vi "Extended Peripherals_labserver_ed.vi"(2 "error in (no error)":errorcluster, 4 "Command In":string) -> (0 "error out (no error)":errorcluster, 1 "DataOut":string)   [LabVIEW 2011]
doc: "Extended Peripherals\n\nThis vi will contain extended functionality not fitting in the regular instrumentation, such as sets and resets.\n\nCommand In:\n0 Delay.\n3 Reset ALL!"
uses:
  Server_Globals.vi
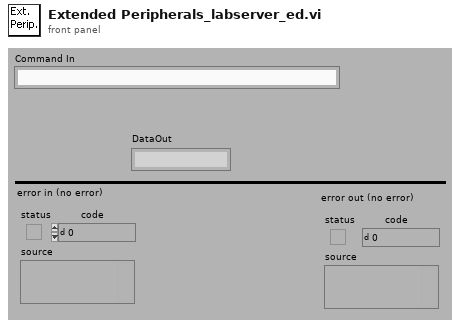
[diagram p1: front panel]
types:
  T1 = cluster{"I/O Settings":u64[], "Instrument Handle":cluster{"5402":refnum<k15>, " 5112":refnum<k15>, "4072":refnum<k15>, "USB":refnum<visa-resource-name>, "4110":refnum<k15>}, "Logfile":refnum<file>, "Log Level":i8, "Clear":i32[], "OS Set":cluster{"instrument handle out":refnum<k15>, "remaining string":string, "Settings":cluster{"Horizontal Conf.":cluster{"Min. Sample rate":dbl, "Reference position":dbl, "Record Length":i16}, "Channel A":cluster{"Enable":bool, "Vertical coupling":dbl, "Vertical range":dbl, "Vertical offset":dbl, "Probe attenuation":dbl}, "Channel B":cluster{"Enable":bool, "Vertical coupling":dbl, "Vertical range":dbl, "Vertical offset":dbl, "Probe attenuation":dbl}, "Trigger":cluster{"Source":enum8{"channel 1", "channel 2", "Imediate", "External trigger"}, "Slope":enum8{"Positive", "Negative"}, "Coupling":enum8{"AC", "DC"}, "Level":dbl, "Holdoff":dbl, "Delay":dbl, " Timeout":dbl, " Mode":enum8{"Normal", "Auto", "Auto Level"}}, "Measurements":cluster{"Measurement 1, Channel":enum8{"Channel 1", "Channel 2", "Channel 3", "Channel 4"}, "Measurement 1, Selection":u16, "Measurement 2, Channel":enum8{"Channel 1", "Channel 2", "Channel 3", "Channel 4"}, "Measurement 2,  Selection":u16, "Measurement 3, Channel":enum8{"Channel 1", "Channel 2", "Channel 3", "Channel 4"}, "Measurement 3, Selection 3":u16}}}, "DC Power Supply":cluster{"0":refnum<k15>, "1":refnum<k15>, "2":refnum<k15>, "3":refnum<k15>, "4":refnum<k15>}, "USB Interface":cluster{"0":refnum<visa-resource-name>, "1":refnum<visa-resource-name>, "2":refnum<visa-resource-name>, "3":refnum<visa-resource-name>, "4":refnum<visa-resource-name>}, "Function Generator":cluster{"0":refnum<k15>, "1":refnum<k15>, "2":refnum<k15>, "3":refnum<k15>, "4":refnum<k15>}, "Digital Multimeter":cluster{"0":refnum<k15>, "1":refnum<k15>, "2":refnum<k15>, "3":refnum<k15>, "4":refnum<k15>}, "Digital Osciliscope":cluster{"0":refnum<k15>, "1":refnum<k15>, "2":refnum<k15>, "3":refnum<k15>, "4":refnum<k15>}, "To M Server":string, "Adres":string[][], "Matrix version":string, "MD5":string, "Digital Multimeter Card 2":cluster{"0":string, "1":string, "2":string, "3":string, "4":string}}
  T2 = cluster{"Global":cluster{"Port":i32, "Reset Time":i32, "Maximum Delay":i32}, "Instrument Adress":cluster{"FGEN":string, "DC Power":string, "OSC":string, "USB":string, "DMM":string}, "Log":cluster{"Log Level":u32, "Log File":path}, "Digital Multimeter":cluster{"0":string, "1":string, "2":string, "3":string, "4":string}, "Function Generator":cluster{"0":string, "1":string, "2":string, "3":string, "4":string}, "Digital Osciliscope":cluster{"0":string, "1":string, "2":string, "3":string, "4":string}, "DC Power Supply":cluster{"0":string, "1":string, "2":string, "3":string, "4":string}, "USB Interface":cluster{"0":string, "1":string, "2":string, "3":string, "4":string}, "Components type":cluster{"Components type":string, "Components list":string}, "Matrix version":string, "Digital Multimeter Card 2":cluster{"0":string, "1":string, "2":string, "3":string, "4":string}}
  T3 = cluster{"0":refnum<k15>, "1":refnum<k15>, "2":refnum<k15>, "3":refnum<k15>, "4":refnum<k15>}
  T4 = cluster{"[0]":refnum<k15>, "[1]":refnum<k15>, "[2]":refnum<k15>, "[3]":refnum<k15>, "[4]":refnum<k15>}
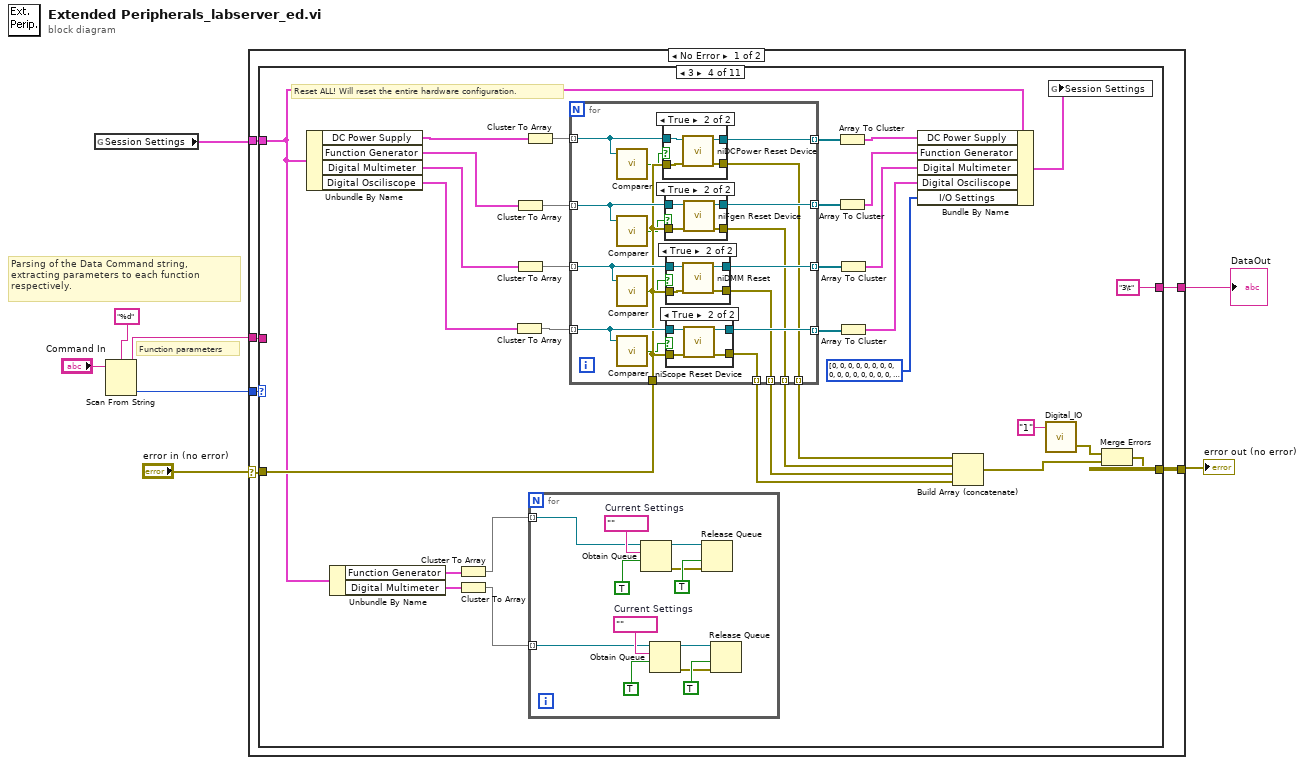
[diagram p0: block diagram]
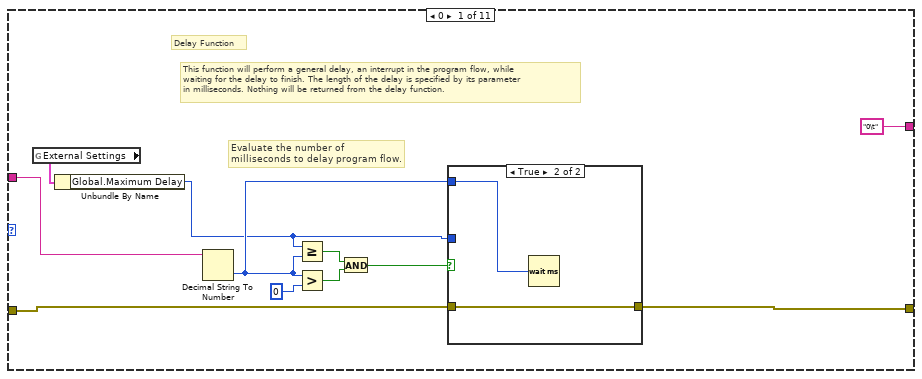
[diagram p2: hidden frame]
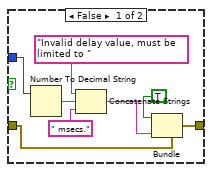
[diagram p3: hidden frame]
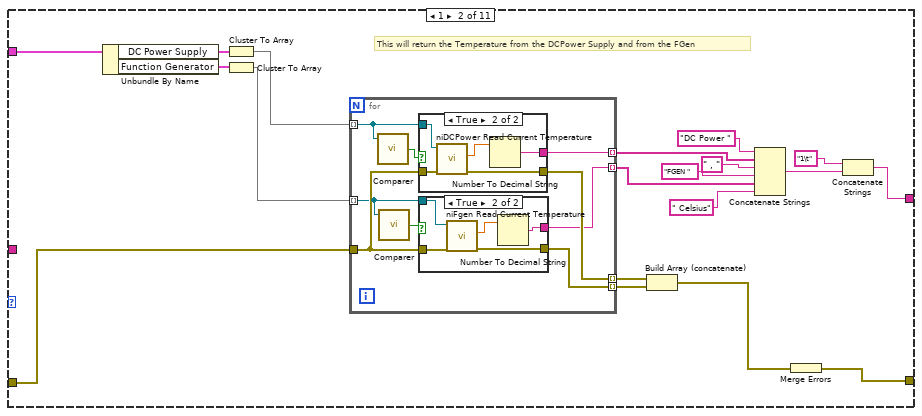
[diagram p4: hidden frame]
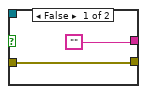
[diagram p5: hidden frame]
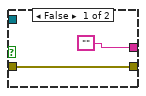
[diagram p6: hidden frame]
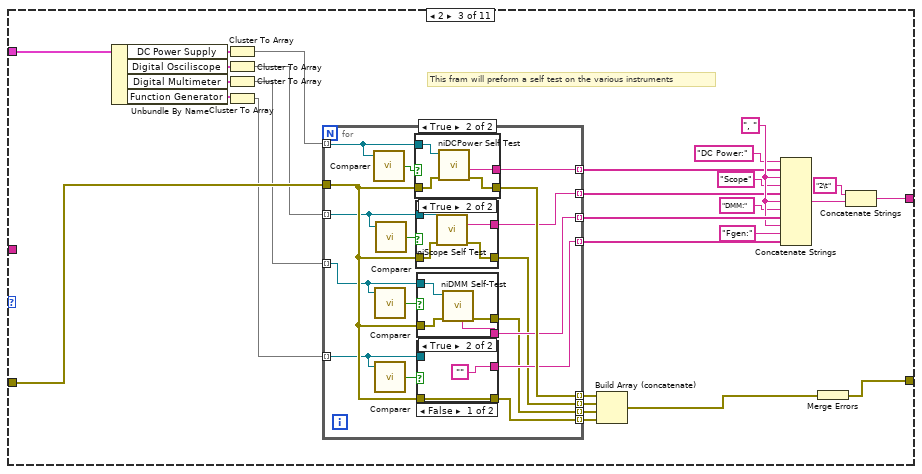
[diagram p7: hidden frame]
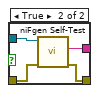
[diagram p8: hidden frame]
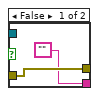
[diagram p9: hidden frame]
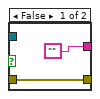
[diagram p10: hidden frame]
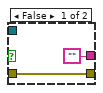
[diagram p11: hidden frame]
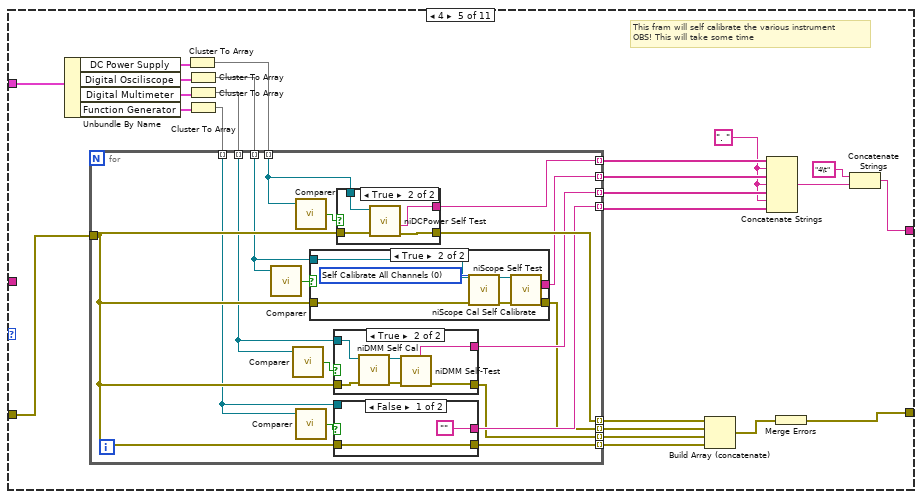
[diagram p16: hidden frame]
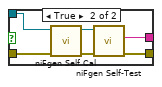
[diagram p17: hidden frame]
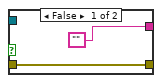
[diagram p18: hidden frame]
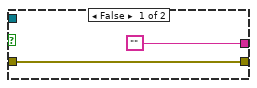
[diagram p19: hidden frame]
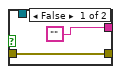
[diagram p20: hidden frame]
diagram:
  # "Function parameters"
  # "Parsing of the Data Command string, extracting parameters to each function respectively."
  n1 = global read "Server_Globals.vi" "Session Settings"() -> (w2:T1)
  n2 = Scan From String(format string="%d", input string="Command In") -> (remaining string=w6:string, output 1=w7:i32)  [unwired: 3 in, 2 out]
  n3 = case shown="No Error" "error in (no error)" {
    selector: "error in (no error)" -> [w11 w555]
    tunnel: w7 -> [w13 _]
    tunnel: w6 -> [w12 _]
    tunnel: [w14 w556] -> w5
    tunnel: w2 -> [w10 _]
    tunnel: [w9 ""] -> w1
    frame No Error {
      n4 = case shown="3" w13 {
        selector: w13 -> [_ _ _ _ _ _ _ _ _ _ w550]
        tunnel: [w20 w53 w78 w179 w233 w305 w370 w409 w473 w483 w549] -> w14
        tunnel: w12 -> [w19 _ _ _ _ _ _ _ _ _ _]
        tunnel: w11 -> [w18 w51 w101 w155 w250 w306 w368 w407 w433 w524 w548]
        tunnel: w10 -> [_ w54 w102 w151 w256 w309 w369 w431 w474 w546 _]
        tunnel: ["0\t" w50 w92 "3\t" w248 "" w347 w420 w449 w484 ""] -> w9
        frame 0 {
          # "This function will perform a general delay, an interrupt in the program flow, while\nwaiting for the delay to finish. The length of the delay is specified by its parameter\nin milliseconds. Nothing will be returned from the delay function."
          # "Evaluate the number of milliseconds to delay program flow."
          # "Delay Function"
          n5 = global read "Server_Globals.vi" "External Settings"() -> (w16:T2)
          n6 = Unbundle By Name(w16) -> ("Global.Maximum Delay"=w15:i32)
          n7 = Decimal String To Number(string=w19) -> (number=w25:i32)  [unwired: 2 in, 1 out]
          n8 = Greater Or Equal?(x=w15, y=w25) -> (x >= y?=w23:bool)
          n9 = Greater?(x=w25, y=0) -> (0:w22:bool)
          n10 = And(x=w23, y=w22) -> (x .and. y?=w24:bool)
          n11 = case shown="True" w24 {
            tunnel: w25 -> [_ w35]
            tunnel: [w26 w34] -> w20
            tunnel: w15 -> [w28 _]
            tunnel: w18 -> [w27 w34]
            frame False {
              n12 = Number To Decimal String(number=w28) -> (decimal integer string=w29:string)  [unwired: 1 in]
              n13 = Concatenate Strings("Invalid delay value, must be limited to " ("source"), w29, " msecs." ("string")) -> (w32:string)
              n14 = Bundle(cluster=w27, "status"=TRUE, "source"=w32) -> (w26:errorcluster)  [unwired: 1 in]
            }
            frame True {
              n15 = Wait (ms)(milliseconds to wait=w35) -> ()  [unwired: 1 out]
            }
          }
        }
        frame 1 {
          # "This will return the Temperature from the DCPower Supply and from the FGen"
          n16 = Unbundle By Name(w54) -> ("DC Power Supply"=w44:T3, "Function Generator"=w42:T3)
          n17 = Cluster To Array(cluster=w44) -> (array=w43:refnum<k15>[])
          n18 = Cluster To Array(cluster=w42) -> (array=w41:refnum<k15>[])
          n19 = for {
            tunnel: w43 -> [w58] mode=indexing
            tunnel: [w63] -> w47 mode=indexing
            tunnel: [w62] -> w39 mode=indexing
            tunnel: [w61] -> w52 mode=indexing
            tunnel: w51 -> [w60]
            tunnel: w41 -> [w57] mode=indexing
            tunnel: [w59] -> w46 mode=indexing
            n20 = call "Comparer.vi"("Resource name"=w58) -> ("Boolean"=w55:bool)  [unwired: 3 in, 1 out]
            n21 = call "Comparer.vi"("Resource name"=w57) -> ("Boolean"=w56:bool)  [unwired: 3 in, 1 out]
            n22 = case shown="True" w55 {
              tunnel: w58 -> [_ w77]
              tunnel: [w71 w76] -> w63
              tunnel: ["" w74] -> w62
              tunnel: w60 -> [w71 w73]
              frame False {
              }
              frame True {
                n23 = call <instrlib>:"niDCPower Read Current Temperature.vi"("error in (no error)"=w73, "instrument handle"=w77) -> ("error out"=w76:errorcluster, "temperature"=w75:dbl)  [unwired: 7 in, 1 out]
                n24 = Number To Decimal String(number=w75) -> (decimal integer string=w74:string)  [unwired: 1 in]
              }
            }
            n25 = case shown="True" w56 {
              tunnel: ["" w70] -> w61
              tunnel: w60 -> [w65 w68]
              tunnel: w57 -> [_ w67]
              tunnel: [w65 w66] -> w59
              frame False {
              }
              frame True {
                n26 = call <instrlib>:"niFgen Read Current Temperature.vi"("error in (no error)"=w68, "Instrument Handle"=w67) -> ("error out"=w66:errorcluster, "Temperature"=w69:dbl)  [unwired: 7 in, 1 out]
                n27 = Number To Decimal String(number=w69) -> (decimal integer string=w70:string)  [unwired: 1 in]
              }
            }
          }
          n28 = Build Array (concatenate)(w47, w46) -> (w45:errorcluster[])
          n29 = Concatenate Strings("DC Power ", w39, " , ", "FGEN ", w52, " Celsius") -> (w49:string)
          n30 = Merge Errors(w45) -> (w53:errorcluster)
          n31 = Concatenate Strings("1\t", w49) -> (w50:string)
        }
        frame 2 {
          w104 = ", "
          # "This fram will preform a self test on the various instruments"
          n32 = Unbundle By Name(w102) -> ("DC Power Supply"=w91:T3, "Digital Osciliscope"=w89:T3, "Digital Multimeter"=w87:T3, "Function Generator"=w84:T3)
          n33 = Cluster To Array(cluster=w91) -> (array=w90:refnum<k15>[])
          n34 = Cluster To Array(cluster=w89) -> (array=w88:refnum<k15>[])
          n35 = Cluster To Array(cluster=w87) -> (array=w86:refnum<k15>[])
          n36 = Cluster To Array(cluster=w84) -> (array=w85:refnum<k15>[])
          n37 = for {
            tunnel: w90 -> [w113] mode=indexing
            tunnel: [w122] -> w83 mode=indexing
            tunnel: [w121] -> w105 mode=indexing
            tunnel: [w120] -> w103 mode=indexing
            tunnel: w88 -> [w112] mode=indexing
            tunnel: w86 -> [w111] mode=indexing
            tunnel: w85 -> [w110] mode=indexing
            tunnel: w101 -> [w119]
            tunnel: [w118] -> w80 mode=indexing
            tunnel: [w117] -> w81 mode=indexing
            tunnel: [w116] -> w82 mode=indexing
            tunnel: [w115] -> w100 mode=indexing
            tunnel: [w114] -> w96 mode=indexing
            n38 = call "Comparer.vi"("Resource name"=w113) -> ("Boolean"=w106:bool)  [unwired: 3 in, 1 out]
            n39 = call "Comparer.vi"("Resource name"=w111) -> ("Boolean"=w108:bool)  [unwired: 3 in, 1 out]
            n40 = call "Comparer.vi"("Resource name"=w110) -> ("Boolean"=w109:bool)  [unwired: 3 in, 1 out]
            n41 = call "Comparer.vi"("Resource name"=w112) -> ("Boolean"=w107:bool)  [unwired: 3 in, 1 out]
            n42 = case shown="True" w106 {
              tunnel: w113 -> [_ w146]
              tunnel: [w142 w145] -> w122
              tunnel: w119 -> [w142 w144]
              tunnel: ["" w143] -> w115
              frame False {
              }
              frame True {
                n43 = call <instrlib>:"niDCPower Self Test.vi"("error in (no error)"=w144, "instrument handle"=w146) -> ("error out"=w145:errorcluster, "self test message"=w143:string)  [unwired: 6 in, 2 out]
              }
            }
            n44 = case shown="True" w107 {
              tunnel: w112 -> [_ w140]
              tunnel: w119 -> [w136 w139]
              tunnel: [w136 w138] -> w116
              tunnel: ["" w137] -> w114
              frame False {
              }
              frame True {
                n45 = call <instrlib>:"niScope Self Test.vi"("instrument handle"=w140, "error in"=w139) -> ("self-test message"=w137:string, "error out"=w138:errorcluster)  [unwired: 10 in, 2 out]
              }
            }
            n46 = case shown="True" w108 {
              tunnel: ["" w134] -> w121
              tunnel: w111 -> [_ w133]
              tunnel: w119 -> [w130 w132]
              tunnel: [w130 w131] -> w117
              frame False {
              }
              frame True {
                n47 = call <instrlib>:"niDMM Self-Test.vi"("error in (no error)"=w132, "instrument handle"=w133) -> ("error out"=w131:errorcluster, "Self Test Message"=w134:string)  [unwired: 6 in, 2 out]
              }
            }
            n48 = case shown="False" w109 {
              tunnel: ["" w128] -> w120
              tunnel: w110 -> [_ w127]
              tunnel: w119 -> [w123 w126]
              tunnel: [w123 w125] -> w118
              frame False {
              }
              frame True {
                n49 = call <instrlib>:"niFgen Self-Test.vi"("error in (no error)"=w126, "Instrument Handle"=w127) -> ("error out"=w125:errorcluster, "Self-Test Message"=w128:string)  [unwired: 6 in, 2 out]
              }
            }
          }
          n50 = Build Array (concatenate)(w83, w82, w81, w80) -> (w79:errorcluster[])
          n51 = Concatenate Strings("DC Power:", w100, w104, "Scope", w96, w104, "DMM:", w105, w104, "Fgen:", w103) -> (w94:string)
          n52 = Merge Errors(w79) -> (w78:errorcluster)
          n53 = Concatenate Strings("2\t", w94) -> (w92:string)
        }
        frame 3 {
          # "Reset ALL! Will reset the entire hardware configuration."
          n54 = Unbundle By Name(w151) -> ("DC Power Supply"=w167:T3, "Function Generator"=w164:T3, "Digital Multimeter"=w165:T3, "Digital Osciliscope"=w166:T3)
          n55 = Unbundle By Name(w151) -> ("Function Generator"=w150:T3, "Digital Multimeter"=w149:T3)
          n56 = Cluster To Array(cluster=w150) -> (array=w148:refnum<k15>[])
          n57 = Cluster To Array(cluster=w149) -> (array=w147:refnum<k15>[])
          n58 = Cluster To Array(cluster=w166) -> (array=w169:refnum<k15>[])
          n59 = Cluster To Array(cluster=w164) -> (array=w173:refnum<k15>[])
          n60 = Cluster To Array(cluster=w165) -> (array=w171:refnum<k15>[])
          n61 = Cluster To Array(cluster=w167) -> (array=w175:refnum<k15>[])
          n62 = for {
            tunnel: w148 -> [w181] mode=indexing
            tunnel: w147 -> [w180] mode=indexing
            w186 = ""  # Current Settings
            w191 = ""  # Current Settings
            n63 = Obtain Queue(name (unnamed)=w181, element data type=w186, create if not found? (T)=TRUE) -> (queue out=w183:refnum<queue>, error out=w184:errorcluster)  [unwired: 2 in, 1 out]
            n64 = Obtain Queue(name (unnamed)=w180, element data type=w191, create if not found? (T)=TRUE) -> (queue out=w188:refnum<queue>, error out=w189:errorcluster)  [unwired: 2 in, 1 out]
            n65 = Release Queue(queue=w183, force destroy? (F)=TRUE, error in (no error)=w184) -> ()  [unwired: 3 out]
            n66 = Release Queue(queue=w188, force destroy? (F)=TRUE, error in (no error)=w189) -> ()  [unwired: 3 out]
          }
          n67 = for {
            tunnel: w175 -> [w204] mode=indexing
            tunnel: [w208] -> w174 mode=indexing
            tunnel: w173 -> [w203] mode=indexing
            tunnel: [w206] -> w172 mode=indexing
            tunnel: w171 -> [w202] mode=indexing
            tunnel: [w207] -> w170 mode=indexing
            tunnel: w169 -> [w201] mode=indexing
            tunnel: [w205] -> w168 mode=indexing
            tunnel: [w200] -> w159 mode=indexing
            tunnel: [w199] -> w158 mode=indexing
            tunnel: [w198] -> w157 mode=indexing
            tunnel: [w197] -> w156 mode=indexing
            tunnel: w155 -> [w196]
            n68 = call "Comparer.vi"("Resource name"=w204) -> ("Boolean"=w192:bool)  [unwired: 3 in, 1 out]
            n69 = call "Comparer.vi"("Resource name"=w203) -> ("Boolean"=w193:bool)  [unwired: 3 in, 1 out]
            n70 = call "Comparer.vi"("Resource name"=w202) -> ("Boolean"=w194:bool)  [unwired: 3 in, 1 out]
            n71 = call "Comparer.vi"("Resource name"=w201) -> ("Boolean"=w195:bool)  [unwired: 3 in, 1 out]
            n72 = case shown="True" w192 {
              tunnel: [w228 w232] -> w208
              tunnel: w204 -> [w228 w231]
              tunnel: [w227 w230] -> w200
              tunnel: w196 -> [w227 w229]
              frame False {
              }
              frame True {
                n73 = call <instrlib>:"niDCPower Reset Device.vi"("error in (no error)"=w229, "instrument handle"=w231) -> ("error out"=w230:errorcluster, "instrument handle out"=w232:refnum<k15>)  [unwired: 8 in]
              }
            }
            n74 = case shown="True" w193 {
              tunnel: w203 -> [w222 w226]
              tunnel: [w222 w225] -> w206
              tunnel: [w221 w224] -> w199
              tunnel: w196 -> [w221 w223]
              frame False {
              }
              frame True {
                n75 = call <instrlib>:"niFgen Reset Device.vi"("error in (no error)"=w223, "Instrument Handle"=w226) -> ("error out"=w224:errorcluster, "Instrument Handle Out"=w225:refnum<k15>)  [unwired: 8 in]
              }
            }
            n76 = case shown="True" w194 {
              tunnel: w202 -> [w216 w220]
              tunnel: [w216 w219] -> w207
              tunnel: [w215 w218] -> w198
              tunnel: w196 -> [w215 w217]
              frame False {
              }
              frame True {
                n77 = call <instrlib>:"niDMM Reset.vi"("error in (no error)"=w217, "instrument handle"=w220) -> ("error out"=w218:errorcluster, "instrument handle out"=w219:refnum<k15>)  [unwired: 8 in]
              }
            }
            n78 = case shown="True" w195 {
              tunnel: w201 -> [w210 w214]
              tunnel: [w210 w213] -> w205
              tunnel: [w209 w212] -> w197
              tunnel: w196 -> [w209 w211]
              frame False {
              }
              frame True {
                n79 = call <instrlib>:"niScope Reset Device.vi"("instrument handle"=w214, "error in"=w211) -> ("instrument handle out"=w213:refnum<k15>, "error out"=w212:errorcluster)  [unwired: 12 in]
              }
            }
          }
          n80 = Array To Cluster(array=w174) -> (cluster=w163:T4)
          n81 = Array To Cluster(array=w172) -> (cluster=w162:T4)
          n82 = Array To Cluster(array=w170) -> (cluster=w161:T4)
          n83 = Array To Cluster(array=w168) -> (cluster=w160:T4)
          n84 = Bundle By Name(cluster=w151, "DC Power Supply"=w163, "Function Generator"=w162, "Digital Multimeter"=w161, "Digital Osciliscope"=w160, "I/O Settings"=i32[] [0, 0, 0, 0, 0, 0, 0, 0, 0, 0, 0, 0, 0, 0, 0, 0, 0, 0, 0, 0, 0, 0, 0, 0, 0, 0, 0, 0, 0, 0, 0, 0]) -> (w176:T1)
          n85 = Build Array (concatenate)(w159, w158, w157, w156) -> (w152:errorcluster[])
          n86 = call "Digital_IO.vi"("Data in"="1") -> ("error out (no error)"=w153:errorcluster)  [unwired: 2 in]
          n87 = global write "Server_Globals.vi" "Session Settings"(w176) -> ()
          n88 = Merge Errors(w153, w152) -> (w179:errorcluster)
        }
        frame 4 {
          w252 = ". "
          # "This fram will self calibrate the various instrument\nOBS! This will take some time"
          n89 = Unbundle By Name(w256) -> ("DC Power Supply"=w246:T3, "Digital Osciliscope"=w244:T3, "Digital Multimeter"=w242:T3, "Function Generator"=w240:T3)
          n90 = Cluster To Array(cluster=w246) -> (array=w245:refnum<k15>[])
          n91 = Cluster To Array(cluster=w244) -> (array=w243:refnum<k15>[])
          n92 = Cluster To Array(cluster=w242) -> (array=w241:refnum<k15>[])
          n93 = Cluster To Array(cluster=w240) -> (array=w239:refnum<k15>[])
          n94 = for {
            tunnel: w245 -> [w264] mode=indexing
            tunnel: [w273] -> w238 mode=indexing
            tunnel: [w272] -> w255 mode=indexing
            tunnel: [w271] -> w254 mode=indexing
            tunnel: [w270] -> w253 mode=indexing
            tunnel: [w269] -> w251 mode=indexing
            tunnel: w243 -> [w263] mode=indexing
            tunnel: w241 -> [w262] mode=indexing
            tunnel: w239 -> [w261] mode=indexing
            tunnel: w250 -> [w268]
            tunnel: [w267] -> w235 mode=indexing
            tunnel: [w266] -> w236 mode=indexing
            tunnel: [w265] -> w237 mode=indexing
            n95 = call "Comparer.vi"("Resource name"=w263) -> ("Boolean"=w258:bool)  [unwired: 3 in, 1 out]
            n96 = call "Comparer.vi"("Resource name"=w262) -> ("Boolean"=w259:bool)  [unwired: 3 in, 1 out]
            n97 = call "Comparer.vi"("Resource name"=w264) -> ("Boolean"=w257:bool)  [unwired: 3 in, 1 out]
            n98 = call "Comparer.vi"("Resource name"=w261) -> ("Boolean"=w260:bool)  [unwired: 3 in, 1 out]
            n99 = case shown="True" w258 {
              tunnel: ["" w295] -> w271
              tunnel: w263 -> [_ w294]
              tunnel: w268 -> [w291 w293]
              tunnel: [w291 w292] -> w265
              frame False {
              }
              frame True {
                w298 = 0 items=["Self Calibrate All Channels", "Restore External Calibration"] ("Option")
                n100 = call <instrlib>:"niScope Cal Self Calibrate.vi"("instrument handle"=w294, "Option"=w298, "error in"=w293) -> ("instrument handle out"=w297:refnum<k15>, "error out"=w296:errorcluster)  [unwired: 11 in]
                n101 = call <instrlib>:"niScope Self Test.vi"("instrument handle"=w297, "error in"=w296) -> ("self-test message"=w295:string, "error out"=w292:errorcluster)  [unwired: 10 in, 2 out]
              }
            }
            n102 = case shown="True" w259 {
              tunnel: ["" w287] -> w270
              tunnel: w262 -> [_ w286]
              tunnel: w268 -> [w283 w285]
              tunnel: [w283 w284] -> w266
              frame False {
              }
              frame True {
                n103 = call <instrlib>:"niDMM Self Cal.vi"("error in (no error)"=w285, "instrument handle"=w286) -> ("error out"=w288:errorcluster, "instrument handle out"=w289:refnum<k15>)  [unwired: 8 in]
                n104 = call <instrlib>:"niDMM Self-Test.vi"("error in (no error)"=w288, "instrument handle"=w289) -> ("error out"=w284:errorcluster, "Self Test Message"=w287:string)  [unwired: 6 in, 2 out]
              }
            }
            n105 = case shown="False" w260 {
              tunnel: ["" w279] -> w269
              tunnel: w261 -> [_ w278]
              tunnel: w268 -> [w275 w277]
              tunnel: [w275 w276] -> w267
              frame False {
              }
              frame True {
                n106 = call <instrlib>:"niFgen Self Cal.vi"("error in (no error)"=w277, "Instrument Handle"=w278) -> ("error out"=w280:errorcluster, "Instrument Handle Out"=w281:refnum<k15>)  [unwired: 8 in]
                n107 = call <instrlib>:"niFgen Self-Test.vi"("error in (no error)"=w280, "Instrument Handle"=w281) -> ("error out"=w276:errorcluster, "Self-Test Message"=w279:string)  [unwired: 6 in, 2 out]
              }
            }
            n108 = case shown="True" w257 {
              tunnel: [w300 w304] -> w273
              tunnel: ["" w303] -> w272
              tunnel: w268 -> [w300 w302]
              tunnel: w264 -> [_ w301]
              frame False {
              }
              frame True {
                n109 = call <instrlib>:"niDCPower Self Test.vi"("error in (no error)"=w302, "instrument handle"=w301) -> ("error out"=w304:errorcluster, "self test message"=w303:string)  [unwired: 6 in, 2 out]
              }
            }
          }
          n110 = Build Array (concatenate)(w238, w237, w236, w235) -> (w234:errorcluster[])
          n111 = Concatenate Strings(w255, w252, w254, w252, w253, w252, w251) -> (w249:string)
          n112 = Merge Errors(w234) -> (w233:errorcluster)
          n113 = Concatenate Strings("4\t", w249) -> (w248:string)
        }
        frame 5 {
          # "Do not use!\nThis is a test fram for closing the USB connection without closing the server"
          n114 = Unbundle By Name(w309) -> ("Instrument Handle.USB"=w307:refnum<visa-resource-name>)
          n115 = call "USBClose.vi"("error in (no error)"=w306, "USB"=w307) -> ("error out"=w305:errorcluster)  [unwired: 9 in]
        }
        frame 6 {
          n116 = Unbundle By Name(w369) -> ("Instrument Handle.5112"=w406:refnum<k15>)
          n117 = property class="niScope"(reference=w406, error in=w368) -> (reference out=w314:refnum<k15>, error out=w370:errorcluster, "Min Sample Rate"=w398:dbl, "Reference Position"=w397:dbl, "Min Number of Points"=w395:i32, "Trigger Source"=w393:string, "Trigger Slope"=w375:i32, "Trigger Coupling"=w373:i32, "Trigger Level"=w379:dbl, "Trigger Holdoff"=w378:dbl, "Trigger Delay"=w377:dbl, "Trigger Type"=w371:i32)
          n118 = Decrement(x=w371) -> (x-1=w372:i32)
          n119 = Decrement(x=w375) -> (x-1=w376:i32)
          n120 = Decrement(x=w373) -> (x-1=w374:i32)
          n121 = Number To Decimal String(number=w372) -> (decimal integer string=w310:string)  [unwired: 1 in]
          n122 = Number To Decimal String(number=w374) -> (decimal integer string=w389:string)  [unwired: 1 in]
          n123 = Format Into String(initial string="", w379) -> (resulting string=w382:string)  [unwired: 2 in, 1 out]
          n124 = Format Into String(initial string="", w378) -> (resulting string=w380:string)  [unwired: 2 in, 1 out]
          n125 = Format Into String(initial string="", w377) -> (resulting string=w384:string)  [unwired: 2 in, 1 out]
          n126 = Format Into String(initial string="", w397) -> (resulting string=w399:string)  [unwired: 2 in, 1 out]
          n127 = Number To Decimal String(number=w395) -> (decimal integer string=w396:string)  [unwired: 1 in]
          n128 = Number To Decimal String(number=w376) -> (decimal integer string=w390:string)  [unwired: 1 in]
          n129 = Format Into String(initial string="", w398) -> (resulting string=w401:string)  [unwired: 2 in, 1 out]
          n130 = Concatenate Strings(w389, " ") -> (w351:string)
          n131 = Concatenate Strings(w399, " ") -> (w355:string)
          n132 = Concatenate Strings(w396, " ") -> (w354:string)
          n133 = Concatenate Strings(w393, " ") -> (w353:string)
          n134 = Concatenate Strings(w390, " ") -> (w352:string)
          n135 = Concatenate Strings(w382, " ") -> (w350:string)
          n136 = Concatenate Strings(w380, " ") -> (w349:string)
          n137 = Concatenate Strings(w401, " ") -> (w356:string)
          n138 = Concatenate Strings(w384, " ") -> (w348:string)
          n139 = Concatenate Strings(w356, w355, w354) -> (w346:string)
          n140 = Concatenate Strings(w353, w352, w351, w350, w349, w348, w310) -> (w323:string)
          n141 = property class="niScope"(reference=w314, "Active Channel"="0") -> ("Vertical Coupling"=w322:i32, "Vertical Range"=w321:dbl, "Vertical Offset"=w320:dbl, "Probe Attenuation"=w319:dbl)  [unwired: 1 in, 2 out]
          n142 = property class="niScope"(reference=w314, "Active Channel"="1") -> ("Vertical Coupling"=w318:i32, "Vertical Range"=w317:dbl, "Vertical Offset"=w316:dbl, "Probe Attenuation"=w315:dbl)  [unwired: 1 in, 2 out]
          n143 = Decrement(x=w318) -> (x-1=w334:i32)
          n144 = Decrement(x=w322) -> (x-1=w357:i32)
          n145 = Format Into String(initial string="", w317) -> (resulting string=w337:string)  [unwired: 2 in, 1 out]
          n146 = Format Into String(initial string="", w316) -> (resulting string=w335:string)  [unwired: 2 in, 1 out]
          n147 = Format Into String(initial string="", w315) -> (resulting string=w340:string)  [unwired: 2 in, 1 out]
          n148 = Format Into String(initial string="", w321) -> (resulting string=w360:string)  [unwired: 2 in, 1 out]
          n149 = Format Into String(initial string="", w320) -> (resulting string=w358:string)  [unwired: 2 in, 1 out]
          n150 = Format Into String(initial string="", w319) -> (resulting string=w363:string)  [unwired: 2 in, 1 out]
          n151 = Number To Decimal String(number=w334) -> (decimal integer string=w339:string)  [unwired: 1 in]
          n152 = Number To Decimal String(number=w357) -> (decimal integer string=w362:string)  [unwired: 1 in]
          n153 = Concatenate Strings(w339, " ") -> (w329:string)
          n154 = Concatenate Strings(w337, " ") -> (w328:string)
          n155 = Concatenate Strings(w335, " ") -> (w327:string)
          n156 = Concatenate Strings(w362, " ") -> (w333:string)
          n157 = Concatenate Strings(w360, " ") -> (w332:string)
          n158 = Concatenate Strings(w358, " ") -> (w331:string)
          n159 = Concatenate Strings(w340, " ") -> (w326:string)
          n160 = Concatenate Strings(w363, " ") -> (w330:string)
          n161 = Concatenate Strings(w333, w332, w331, w330) -> (w325:string)
          n162 = Concatenate Strings(w329, w328, w327, w326) -> (w324:string)
          n163 = Concatenate Strings(w346, w325, w324, w323) -> (w347:string)
        }
        frame 7 {
          n164 = Unbundle By Name(w431) -> ("Instrument Handle.4072"=w408:refnum<k15>)
          n165 = property class="niDMM"(reference=w408, error in=w407) -> (error out=w409:errorcluster, "Function"=w419:i32, "Digits Resolution"=w417:dbl, "Auto Range Value"=w413:dbl, "Absolute Resolution"=w411:dbl)  [unwired: 1 out]
          n166 = Decrement(x=w419) -> (x-1=w430:i32)
          n167 = Format Into String(initial string="", w411) -> (resulting string=w410:string)  [unwired: 2 in, 1 out]
          n168 = Format Into String(initial string="", w417) -> (resulting string=w414:string)  [unwired: 2 in, 1 out]
          n169 = Format Into String(initial string="", w413) -> (resulting string=w412:string)  [unwired: 2 in, 1 out]
          n170 = Number To Decimal String(number=w430) -> (decimal integer string=w429:string)  [unwired: 1 in]
          n171 = Concatenate Strings(w429, " ") -> (w427:string)
          n172 = Concatenate Strings(w414, " ") -> (w425:string)
          n173 = Concatenate Strings(w412, " ") -> (w423:string)
          n174 = Concatenate Strings(w410, " ") -> (w421:string)
          n175 = Concatenate Strings(w427, w425, w423, w421) -> (w420:string)
        }
        frame 8 {
          n176 = Unbundle By Name(w474) -> ("Instrument Handle.5402"=w432:refnum<k15>)
          n177 = property class="niFgen"(reference=w432, error in=w433) -> (error out=w473:errorcluster, "Waveform"=w469:i32, "Amplitude"=w448:dbl, "Frequency"=w443:dbl, "DC Offset"=w440:dbl, "Start Phase"=w438:dbl, "Trigger Mode"=w459:i32, "Trigger Source"=w458:i32, "Duty Cycle High"=w434:dbl)  [unwired: 1 out]
          n178 = Decrement(x=w469) -> (x-1=w472:i32)
          n179 = Format Into String(initial string="", w438) -> (resulting string=w437:string)  [unwired: 2 in, 1 out]
          n180 = Number To Decimal String(number=w472) -> (decimal integer string=w471:string)  [unwired: 1 in]
          n181 = Format Into String(initial string="", w443) -> (resulting string=w444:string)  [unwired: 2 in, 1 out]
          n182 = Format Into String(initial string="", w440) -> (resulting string=w441:string)  [unwired: 2 in, 1 out]
          n183 = Number To Decimal String(number=w459) -> (decimal integer string=w463:string)  [unwired: 1 in]
          n184 = Number To Decimal String(number=w458) -> (decimal integer string=w461:string)  [unwired: 1 in]
          n185 = Format Into String(initial string="", w448) -> (resulting string=w446:string)  [unwired: 2 in, 1 out]
          n186 = Format Into String(initial string="", w434) -> (resulting string=w435:string)  [unwired: 2 in, 1 out]
          n187 = Concatenate Strings(w471, " ") -> (w457:string)
          n188 = Concatenate Strings(w446, " ") -> (w456:string)
          n189 = Concatenate Strings(w444, " ") -> (w455:string)
          n190 = Concatenate Strings(w441, " ") -> (w454:string)
          n191 = Concatenate Strings(w435, " ") -> (w450:string)
          n192 = Concatenate Strings(w437, " ") -> (w453:string)
          n193 = Concatenate Strings(w463, " ") -> (w452:string)
          n194 = Concatenate Strings(w461, " ") -> (w451:string)
          n195 = Concatenate Strings(w457, w456, w455, w454, w453, w452, w451, w450) -> (w449:string)
        }
        frame 9 {
          n196 = Unbundle By Name(w546) -> ("Instrument Handle.5112"=w545:refnum<k15>)
          n197 = property class="niScope"(reference=w545, error in=w524) -> (error out=w483:errorcluster, "Min Sample Rate"=w523:dbl, "Reference Position"=w522:dbl, "Min Number of Points"=w520:i32, "Vertical Coupling"=w475:i32, "Vertical Range"=w516:dbl, "Vertical Offset"=w513:dbl, "Probe Attenuation"=w512:dbl, "Trigger Source"=w510:string, "Trigger Slope"=w480:i32, "Trigger Coupling"=w478:i32, "Trigger Level"=w493:dbl, "Trigger Holdoff"=w492:dbl, "Trigger Delay"=w491:dbl, "Trigger Type"=w476:i32)  [unwired: 1 out]
          n198 = Decrement(x=w480) -> (x-1=w481:i32)
          n199 = Decrement(x=w478) -> (x-1=w479:i32)
          n200 = Decrement(x=w476) -> (x-1=w477:i32)
          n201 = Decrement(x=w475) -> (x-1=w482:i32)
          n202 = Format Into String(initial string="", w516) -> (resulting string=w517:string)  [unwired: 2 in, 1 out]
          n203 = Format Into String(initial string="", w513) -> (resulting string=w514:string)  [unwired: 2 in, 1 out]
          n204 = Format Into String(initial string="", w512) -> (resulting string=w525:string)  [unwired: 2 in, 1 out]
          n205 = Number To Decimal String(number=w477) -> (decimal integer string=w490:string)  [unwired: 1 in]
          n206 = Number To Decimal String(number=w482) -> (decimal integer string=w519:string)  [unwired: 1 in]
          n207 = Number To Decimal String(number=w479) -> (decimal integer string=w505:string)  [unwired: 1 in]
          n208 = Format Into String(initial string="", w493) -> (resulting string=w496:string)  [unwired: 2 in, 1 out]
          n209 = Format Into String(initial string="", w492) -> (resulting string=w494:string)  [unwired: 2 in, 1 out]
          n210 = Format Into String(initial string="", w491) -> (resulting string=w498:string)  [unwired: 2 in, 1 out]
          n211 = Format Into String(initial string="", w522) -> (resulting string=w527:string)  [unwired: 2 in, 1 out]
          n212 = Number To Decimal String(number=w520) -> (decimal integer string=w521:string)  [unwired: 1 in]
          n213 = Number To Decimal String(number=w481) -> (decimal integer string=w506:string)  [unwired: 1 in]
          n214 = Format Into String(initial string="", w523) -> (resulting string=w529:string)  [unwired: 2 in, 1 out]
          n215 = Concatenate Strings(w490, "") -> (w485:string)
          n216 = Concatenate Strings(w519, "") -> (w534:string)
          n217 = Concatenate Strings(w517, " ") -> (w533:string)
          n218 = Concatenate Strings(w514, " ") -> (w532:string)
          n219 = Concatenate Strings(w505, "") -> (w503:string)
          n220 = Concatenate Strings(w527, " ") -> (w536:string)
          n221 = Concatenate Strings(w521, " ") -> (w535:string)
          n222 = Concatenate Strings(w525, " ") -> (w531:string)
          n223 = Concatenate Strings(w510, " ") -> (w509:string)
          n224 = Concatenate Strings(w506, " ") -> (w504:string)
          n225 = Concatenate Strings(w496, " ") -> (w488:string)
          n226 = Concatenate Strings(w494, " ") -> (w487:string)
          n227 = Concatenate Strings(w529, " ") -> (w537:string)
          n228 = Concatenate Strings(w498, " ") -> (w486:string)
          n229 = Concatenate Strings(w537, w536, w535, w534, w533, w532, w531, w509, w504, w503, w488, w487, w486, w485) -> (w484:string)
        }
        frame Default {
          # "Any other function is ment for the Extra Peripherals and is therefore \nforwarded to that vi."
          n230 = Number To Decimal String(number=w550) -> (decimal integer string=w551:string)  [unwired: 1 in]
          n231 = Concatenate Strings("Extended Peripherals VI reports:\nUnknown command: ", w551) -> (w553:string)
          n232 = Bundle(cluster=w548, "status"=TRUE, "source"=w553) -> (w549:errorcluster)  [unwired: 1 in]
        }
      }
    }
    frame Error {
      # "Errors have occoured!"
      n233 = call "Error Converter.vi"("error in (no error)"=w555, "String to add to error message"="Message from Extended Peripherals:" ("String to add message")) -> ("error out (no error)"=w556:errorcluster)
    }
  }
  "error out (no error)" <- w5
  "DataOut" <- w1
